vi "Initalise.vi"(8 "error in (no error)":errorcluster, 11 "FPGA Interface":refnum<k20>) -> (0 "Encoder Index Position":i16, 2 "Error out":errorcluster, 3 "FPGA VI Reference Out":refnum<k20>)   [LabVIEW 2016]
uses:
  Typedef/INS Data.ctl
  <vilib>/Utility/error.llb/Error Cluster From Error Code.vi
  <vilib>/rvi/errors/niLvFpgaAdjustHostInterfaceError.vi
  <vilib>/rvi/interface/nirviReadWriteControl/nirviReadWriteControl.xnode
  <vilib>/rvi/interface/Simulation/niFpgaSimulationCallBeginRW.vi
  NiFpgaLv.dll
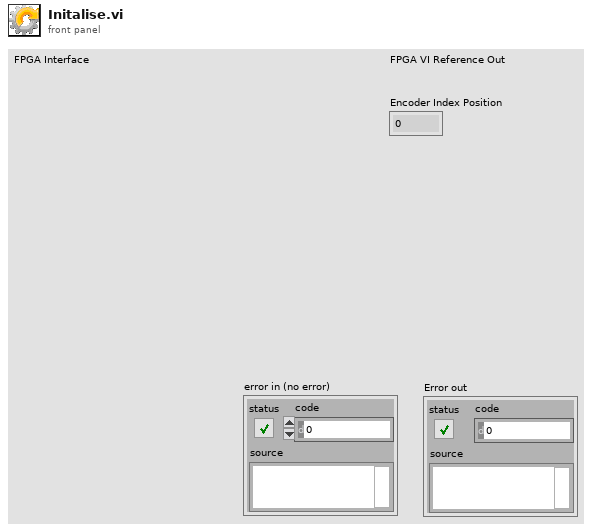
[diagram p1: front panel]
types:
  T1 = typedef "INS Data.ctl" = cluster{"Yaw":sgl, "Pitch":sgl, "Roll":sgl, "Lat":dbl, "Long":dbl, "Alt":dbl, "North":dbl, "East":dbl, "Down":dbl, "PosU":dbl, "VelU":dbl}
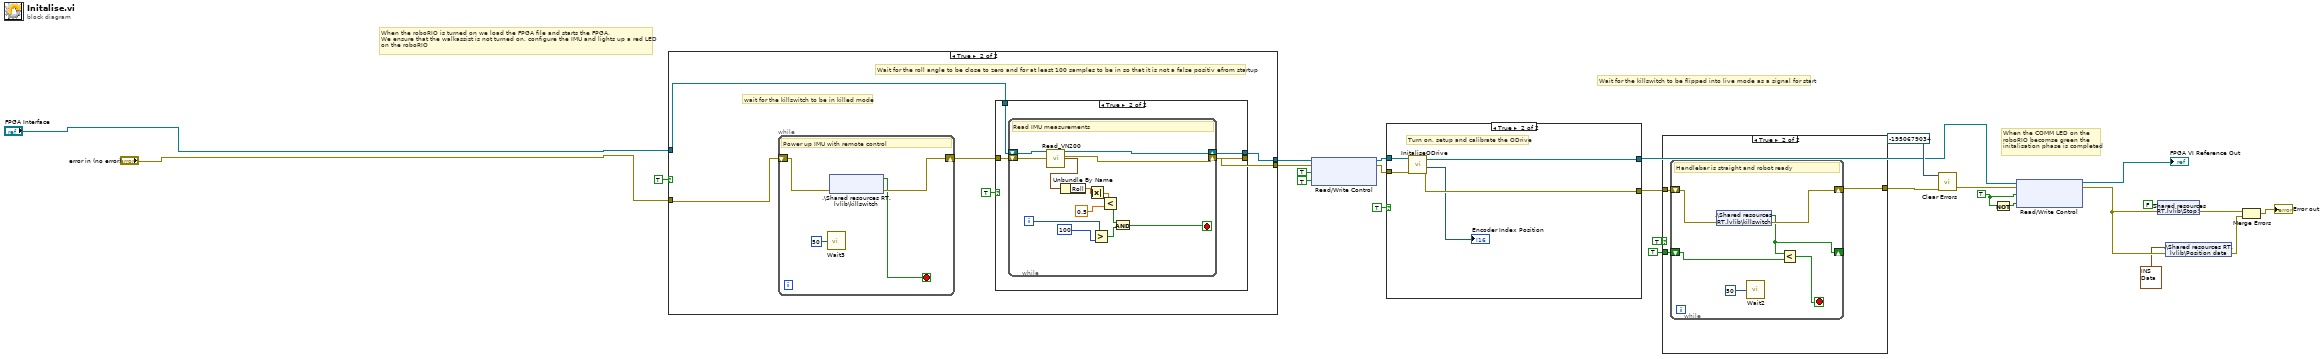
[diagram p0: block diagram]
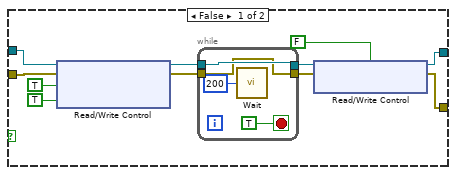
[diagram p5: hidden frame]
diagram:
  w22 = TRUE ("Steering motor on?")
  # "Wait for the killswitch to be flipped into live mode as a signal for start"
  # "When the COMM LED on the\nroboRIO becomse green the\ninitalisation phase is completed"
  # "When the roboRIO is turned on we load the FPGA file and starts the FPGA.\nWe ensure that the walkassist is not turned on, configure the IMU and lights up a red LED\non the roboRIO"
  n1 = case shown="True" TRUE {
    tunnel: "error in (no error)" -> [w27 w29]
    tunnel: "FPGA Interface" -> [w28 w33]
    tunnel: [w28 w32] -> w15
    tunnel: [w27 w31] -> w14
    frame False {
    }
    frame True {
      # "Wait for the roll angle to be close to zero and for at least 100 samples to be in so that it is not a false positiv efrom startup"
      # "wait for the killswitch to be in killed mode"
      n2 = while {
        shift-right: [w56] -> w34
        shift-left: w29 -> [w57]
        stop <- w55 stop-if-true
        # "Power up IMU with remote control"
        n3 = call "Wait3"("Count(mSec)"=u32 50) -> ()  [unwired: 1 out]
        n4 = shared-variable ".\\Shared resources RT.lvlib\\killswitch"(error in=w57) -> (w55:bool, error out=w56:errorcluster)  [unwired: 1 out]
      }
      n5 = case shown="True" TRUE {
        tunnel: w34 -> [w35 w40]
        tunnel: w33 -> [w36 w39]
        tunnel: [w36 w38] -> w32
        tunnel: [w35 w37] -> w31
        frame False {
        }
        frame True {
          n6 = while {
            shift-right: [w50] -> w38
            shift-left: w39 -> [w51]
            shift-right: [w48] -> w37
            shift-left: w40 -> [w49]
            i -> [w52]
            stop <- w53 stop-if-true
            # "Read IMU measurements"
            n7 = call "Read_VN200.vi"("FPGA Interface"=w51, "error in"=w49) -> ("FPGA Interface Out"=w50:refnum<k20>, "error out"=w48:errorcluster, "Position Data"=w45:T1)  [unwired: 11 in]
            n8 = Unbundle By Name(w45) -> ("Roll"=w44:sgl)
            n9 = Absolute Value(x=w44) -> (abs(x)=w43:sgl)
            n10 = Greater?(x=w52, y=100 ("x")) -> (0:w47:bool)
            n11 = Less?(x=w43, y=sgl 0.5) -> (x < y?=w41:bool)
            n12 = And(x=w41, y=w47) -> (x .and. y?=w53:bool)
          }
        }
      }
    }
  }
  n13 = xnode "Read/Write Control"("FPGA VI Reference In"=w15, "error in"=w14, "Comm LED Green"=TRUE, "Comm LED Red"=TRUE) -> ("FPGA VI Reference Out"=w13:refnum<k20>, "error out"=w12:errorcluster)
  n14 = case shown="True" TRUE {
    tunnel: [w59 w77] -> w17
    tunnel: w13 -> [w65 w76]
    tunnel: w12 -> [w66 w75]
    tunnel: [w60 w74] -> w8
    frame False {
      n15 = xnode "Read/Write Control"("FPGA VI Reference In"=w65, "error in"=w66, "ODrive RT Control"=TRUE, "MotorsON"=TRUE) -> ("FPGA VI Reference Out"=w64:refnum<k20>, "error out"=w62:errorcluster)
      n16 = while {
        tunnel: [w70] -> w63
        tunnel: w64 -> [w70]
        tunnel: w62 -> [w69]
        tunnel: [w69] -> w61
        stop <- TRUE stop-if-true
        n17 = call "Wait"("Count(mSec)"=u32 200) -> ()  [unwired: 1 out]
      }
      n18 = xnode "Read/Write Control"("FPGA VI Reference In"=w63, "error in"=w61, "ODrive RT Control"=FALSE) -> ("FPGA VI Reference Out"=w60:refnum<k20>, "error out"=w59:errorcluster)
    }
    frame True {
      # "Turn on, setup and calibrate the ODrive"
      n19 = call "InitaliseODrive.vi"("error in (no error)"=w75, "FPGA Interface in"=w76) -> ("error out"=w77:errorcluster, "Encoder Index Position"=→"Encoder Index Position":i16, "FPGA Interface out"=w74:refnum<k20>)  [unwired: 7 in]
    }
  }
  n20 = case shown="True" TRUE {
    tunnel: w17 -> [w78 w81]
    tunnel: TRUE -> [_ w80]
    tunnel: [w78 w79] -> w9
    frame False {
    }
    frame True {
      n21 = while {
        shift-right: [w86] -> w79
        shift-left: w81 -> [w87]
        shift-right: [w84] -> _
        shift-left: w80 -> [w85]
        stop <- w83 stop-if-true
        # "Handlebar is straight and robot ready"
        n22 = shared-variable ".\\Shared resources RT.lvlib\\killswitch"(error in=w87) -> (w84:bool, error out=w86:errorcluster)
        n23 = call "Wait2"("Count(mSec)"=u32 50) -> ()  [unwired: 1 out]
        n24 = Less?(x=w84, y=w85) -> (x < y?=w83:bool)
      }
    }
  }
  n25 = call <vilib>:"Clear Errors.vi"("error in (no error)"=w9, "specific error code to clear (0: all)"=-1950679034) -> ("error out"=w26:errorcluster)  [unwired: 4 in, 1 out]
  n26 = Not(x=w22) -> (.not. x?=w23:bool)
  n27 = xnode "Read/Write Control"("FPGA VI Reference In"=w8, "error in"=w26, "Comm LED Green"=w22, "Comm LED Red"=w23) -> ("FPGA VI Reference Out"=→"FPGA VI Reference Out":refnum<k20>, "error out"=w21:errorcluster)
  n28 = shared-variable ".\\Shared resources RT.lvlib\\Stop!"(FALSE ("Stop!"), error in=w21) -> (error out=w19:errorcluster)
  n29 = shared-variable ".\\Shared resources RT.lvlib\\Position data"(T1 {"Yaw"=0.0, "Pitch"=0.0, "Roll"=0.0, "Lat"=0.0, "Long"=0.0, "Alt"=0.0, "North"=0.0, "East"=0.0, "Down"=0.0, "PosU"=0.0, "VelU"=0.0} ("Position data"), error in=w21) -> (error out=w18:errorcluster)
  n30 = Merge Errors(w19, w18) -> (→"Error out":errorcluster)
